vi "generate intensity plot data.vi"(7 "Dataset Path":string="s21mag", 8 "error in (no error)":errorcluster, 11 "path":path=path "C:/Users/dvh-collab-user/Desktop/20230313 Robert sample/tmp.hdf5") -> (0 "error out":errorcluster, 2 "Attribute Value(s) out":T1, 3 "Data out":dbl[][](array[numeric]))   [LabVIEW 2021]
uses:
  <vilib>/Utility/miscctls.llb/LVRectTypeDef.ctl
  <vilib>/UPVI/lvhdf5/group.llb/H5G_obj_t.ctl
  <vilib>/UPVI/lvhdf5/file.llb/LVH5F Operation.ctl
  <vilib>/UPVI/lvhdf5/dataset.llb/LVH5D Operation.ctl
  <vilib>/UPVI/lvhdf5/identifier.llb/Not an HDF5 Refnum Constant.vi
  <vilib>/UPVI/lvhdf5/file.llb/H5Fopen.vi
  <vilib>/UPVI/lvhdf5/utility.llb/Select HDF5 Dialog.vi
  <vilib>/UPVI/lvhdf5/utility.llb/Select HDF5 Dialog (File and Object).vi
  <vilib>/UPVI/lvhdf5/dataset.llb/Simple H5Dread (Variant).vi
  <vilib>/UPVI/lvhdf5/attribute.llb/Read Multiple Attributes (Variant).vi
  <vilib>/UPVI/lvhdf5/common.llb/To HDF5 Ref.vi
  <vilib>/UPVI/lvhdf5/dataset.llb/H5Dclose.vi
  <vilib>/Utility/Data Type/Get Cluster Information.vi
  <vilib>/Utility/Data Type/Get Type Information.vi
  <vilib>/UPVI/lvhdf5/dataset.llb/Read Dataset and All Attributes.xnode
  <vilib>/UPVI/lvhdf5/library.llb/HDF5 Ref.ctl
  <vilib>/UPVI/lvhdf5/attribute.llb/Attribute Array to Cluster.xnode
  <vilib>/UPVI/lvhdf5/library.llb/HDF5 Ref.lvclass
  <vilib>/UPVI/lvhdf5/utility.llb/Select HDF5 Dialog (Object Only).vi
  <vilib>/UPVI/lvhdf5/dataset.llb/OpenCreateReplace Dataset.vi
  <vilib>/UPVI/lvhdf5/dataset.llb/H5Dget_space.vi
  <vilib>/UPVI/lvhdf5/dataspace.llb/H5Sget_simple_extent_dims.vi
  <vilib>/UPVI/lvhdf5/dataspace.llb/H5Sselect_hyperslab.vi
  <vilib>/UPVI/lvhdf5/dataset.llb/H5Dread (Variant).vi
  <vilib>/UPVI/lvhdf5/attribute.llb/private/LVH5AreadWDTAttrs.vi
  <vilib>/UPVI/lvhdf5/dataspace.llb/H5Sclose.vi
  <vilib>/Utility/error.llb/Error Cluster From Error Code.vi
  <vilib>/Utility/Data Type/NI_Data Type.lvlib
panel:
  in  "attrs":T1
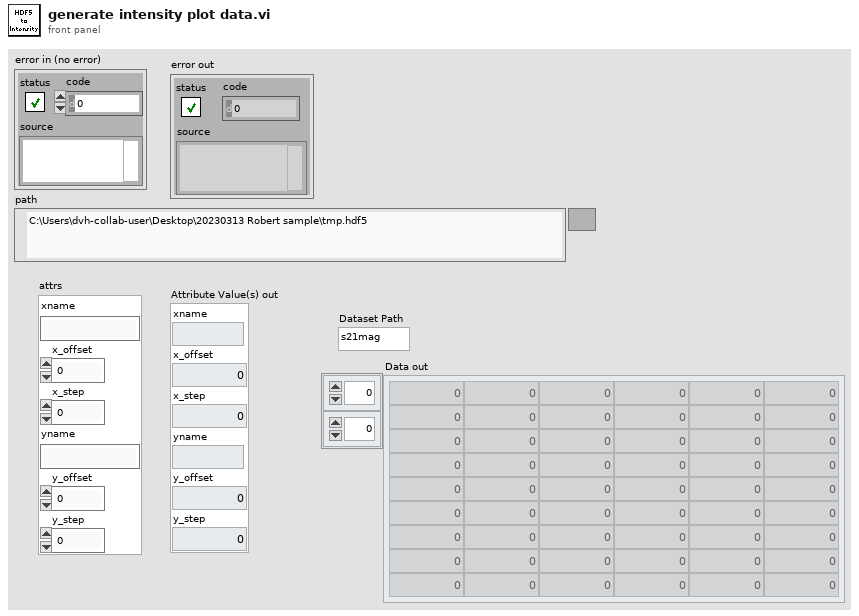
[diagram p1: front panel]
types:
  T1 = cluster{"xname":string, "x_offset":dbl, "x_step":dbl, "yname":string, "y_offset":dbl, "y_step":dbl}
  T2 = typedef "HDF5 Ref.ctl" = refnum<class "HDF5 Ref.lvclass">
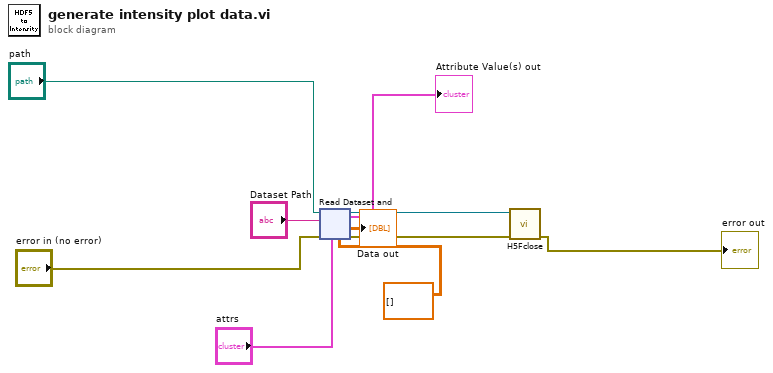
[diagram p0: block diagram]
diagram:
  n1 = xnode "Read Dataset and"("Dataset Path"="Dataset Path", "error in (no error)"="error in (no error)", "HDF5 Path or Ref"="path", "Attribute Value(s)"="attrs", "Data"=dbl[][] []) -> ("HDF5 Ref out"=w6:T2, "error out"=w5:errorcluster, "Attribute Value(s) out"=→"Attribute Value(s) out":T1, "Data out"=→"Data out":dbl[][])  [unwired: 1 in, 2 out]
  n2 = call <vilib>:"H5Fclose.vi"("error in (no error)"=w5, "HDF5 Ref"=w6) -> ("error out"=→"error out":errorcluster)  [unwired: 7 in]
